vi "Sylvester Equations.vi"   [LabVIEW 2020, in "NI_AALPro.lvlib"]
doc: "Solves the Sylvester matrix equation. The data types you wire to the <B>A</B>, <B>B</B>, and <B>C</B> inputs determine the polymorphic instance to use."
uses:
  <vilib>/Analysis/NI_AALPro.lvlib
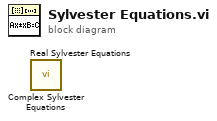
[diagram p0: block diagram]
diagram:
  n1 = call <vilib>:"Complex Sylvester Equations.vi"() -> ()  [unwired: 8 in, 4 out]
  n2 = call <vilib>:"Real Sylvester Equations.vi"() -> ()  [unwired: 8 in, 4 out]
